vi "Dispenser Manual Control.vi"() -> ()   [LabVIEW 2017]
uses:
  Shared Components/Gantry Class/Type Definitions/Init_Modes.ctl
  Shared Components/Gantry Class/Gantry Class.lvclass
panel:
  in  "stop":bool
  in  "Dispenser State":bool
  out "error out":errorcluster
  in  "Config Folder":path=path "C:/Users/Husker/Desktop/gantry/Config"
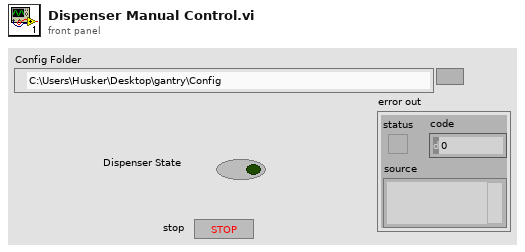
[diagram p1: front panel]
types:
  T1 = typedef "Init_Modes.ctl" = enum16{"Full", "Robot Only", "Dispenser Only", "Cameras Only", "Robot and Cameras", "Robot and Cameras and Dispenser", "Manifold Only"}
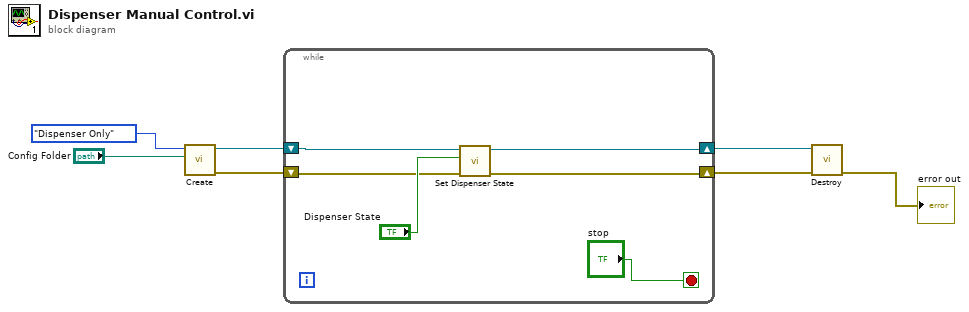
[diagram p0: block diagram]
diagram:
  n1 = call "Create.vi"("Config Folder"="Config Folder", "Init Mode"=Init_Modes."Dispenser Only") -> ("error out"=w1:errorcluster, "Gantry out"=w2:refnum<class "Gantry Class.lvclass">)  [unwired: 8 in]
  n2 = while {
    shift-right: [w9] -> w6
    shift-left: w2 -> [w13]
    shift-right: [w10] -> w5
    shift-left: w1 -> [w11]
    stop <- "stop" stop-if-true
    n3 = call-dynamic "Set Dispenser State.vi"("error in"=w11, "On/Off"="Dispenser State", "Gantry in"=w13) -> ("error out"=w10:errorcluster, "Gantry out"=w9:refnum<class "Gantry Class.lvclass">)  [unwired: 7 in]
  }
  n4 = call "Destroy.vi"("error in"=w5, "Gantry Class in"=w6) -> ("error out"=→"error out":errorcluster)  [unwired: 9 in]
